vi "Vladina provera.vi"() -> ()   [LabVIEW 2012]
uses:
  Globalna_Variabla.vi
panel:
  out "x = y?":bool
  in  "Array":dbl[](array[numeric])
  in  "Reset":bool
  in  "vi path":path=path "C:/Users/Embedded Design/Desktop/Bas Ruten/RS232.vi"
  out "reference out":refnum<vi>
  out "Boolean 2":bool
  in  "stop":bool=TRUE
  out "Sekvenca RS232":dbl[](array[numeric])
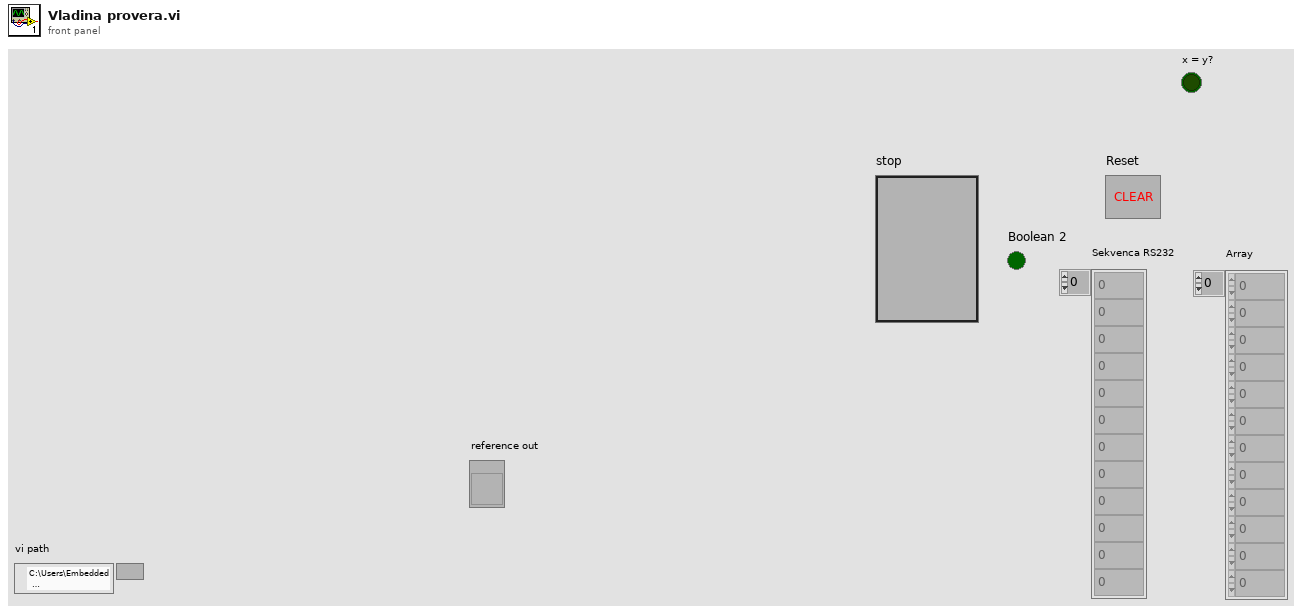
[diagram p1: front panel]
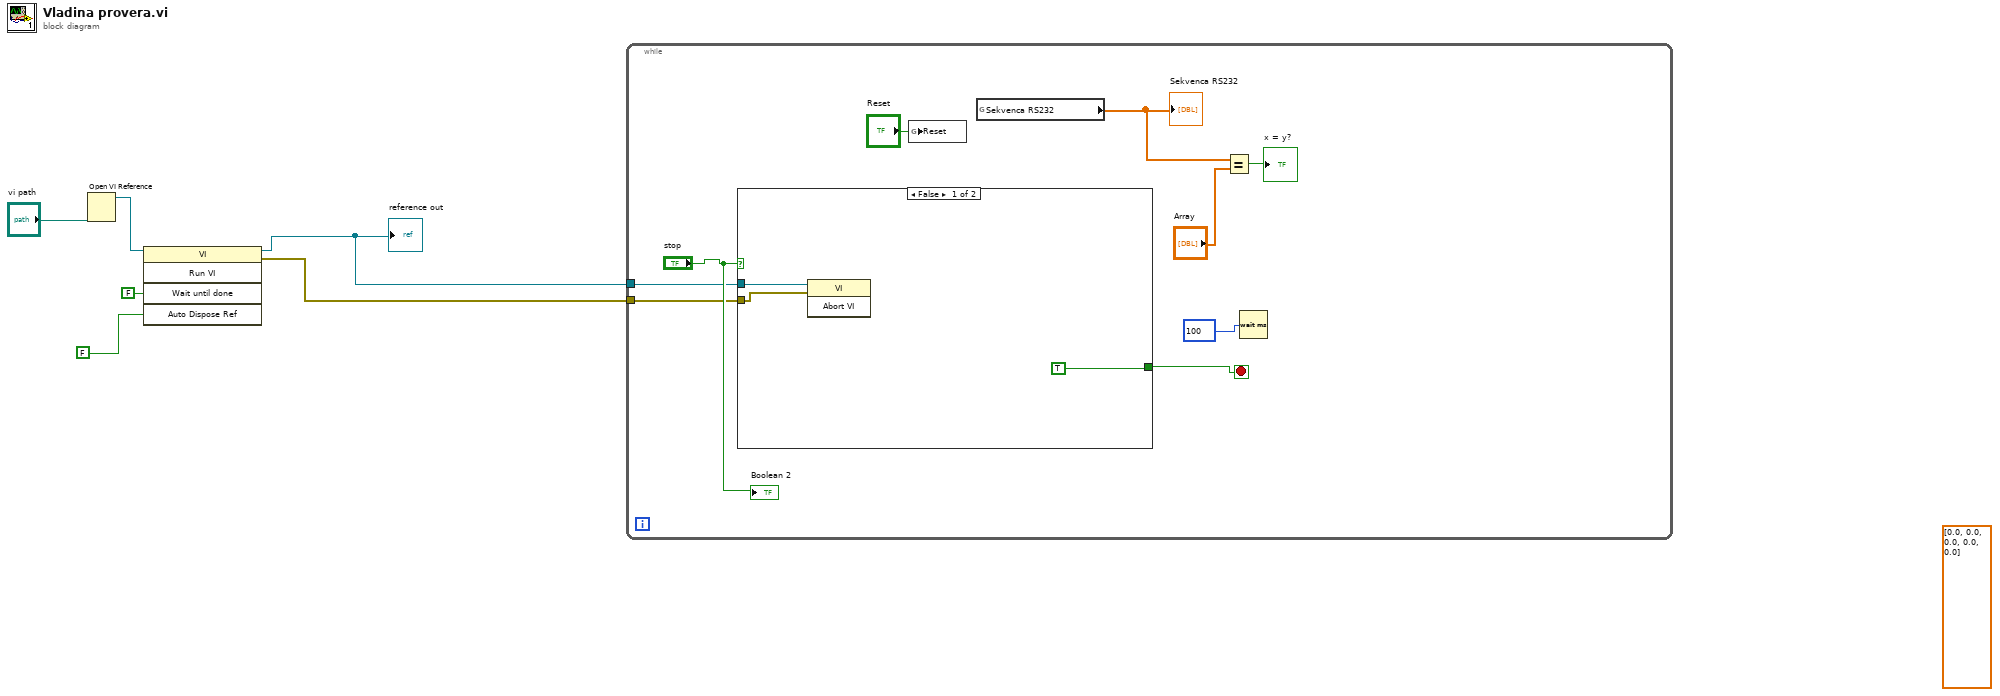
[diagram p0: block diagram]
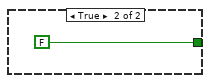
[diagram p2: hidden frame]
diagram:
  (unwired) dbl[] [0.0, 0.0, 0.0, 0.0, 0.0] ("Sekvenca RS232")
  n1 = Open VI Reference(vi path="vi path") -> (vi reference=w5:refnum<vi>)  [unwired: 5 in, 1 out]
  n2 = invoke class="VI" method="Run VI"(reference=w5, "Wait until done"=FALSE ("Wait Until Done"), "Auto Dispose Ref"=FALSE ("Auto Dispose Reference")) -> (reference out=w2:refnum<vi>, error out=w1:errorcluster)  [unwired: 2 in, 3 out]
  "reference out" <- w2
  n3 = while {
    tunnel: w2 -> [w12]
    tunnel: w1 -> [w11]
    stop <- w13 stop-if-true
    n4 = case shown="False" "stop" {
      tunnel: [TRUE FALSE] -> w13
      tunnel: w12 -> [w17 _]
      tunnel: w11 -> [w16 _]
      frame False {
        n5 = invoke class="VI" method="Abort VI"(reference=w17, error in=w16) -> ()  [unwired: 1 in, 3 out]
      }
      frame True {
      }
    }
    n6 = global write "Globalna_Variabla.vi" "Reset"("Reset") -> ()
    n7 = global read "Globalna_Variabla.vi" "Sekvenca RS232"() -> (w9:dbl[])
    "Sekvenca RS232" <- w9
    n8 = Equal?(x=w9, y="Array") -> (x = y?=→"x = y?":bool)
    n9 = Wait (ms)(milliseconds to wait=u32 100) -> ()  [unwired: 1 out]
    "Boolean 2" <- "stop"
  }
